vi "test_leadLag.vi"() -> ()   [LabVIEW 2019]
uses:
  <vilib>/Rock Robotics/WPI/ThirdParty/JAS_Junk/TrajLib/Util_GetTime.vi
  <vilib>/Rock Robotics/WPI/ThirdParty/JAS_Junk/TrajLib/Trajectory_Library.lvlib
panel:
  out "Waveform Chart":cluster{"Slide 2":dbl, "Output":dbl}(graph)
  in  "Lag Time Const (Sec)":dbl
  in  "Lead Time Const (Sec)":dbl
  in  "Enable":bool=TRUE
  out "Output":dbl(slide) scale=0.0..10.0
  in  "Input":dbl(slide) scale=0.0..10.0
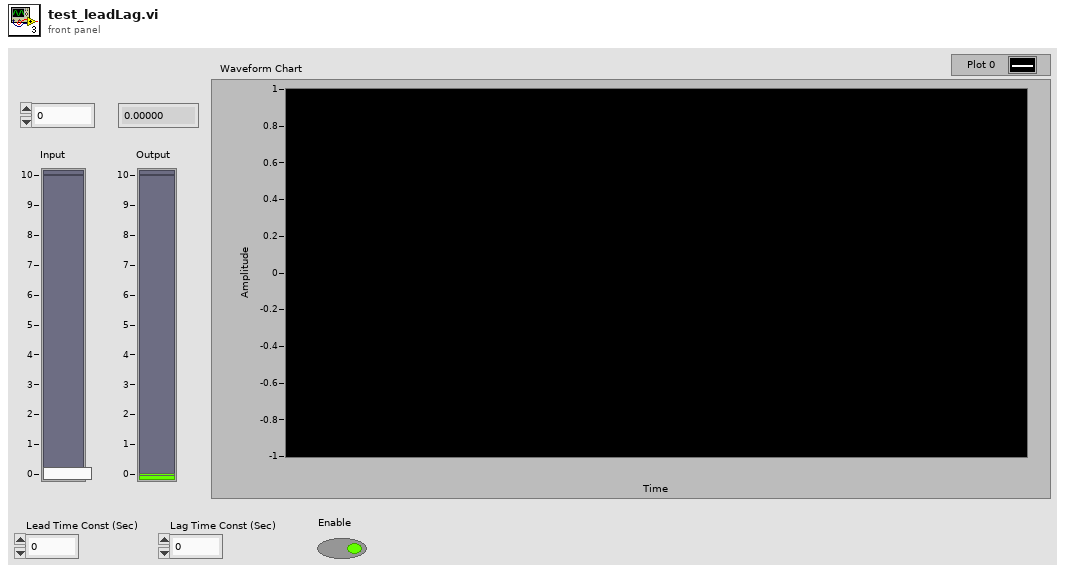
[diagram p1: front panel]
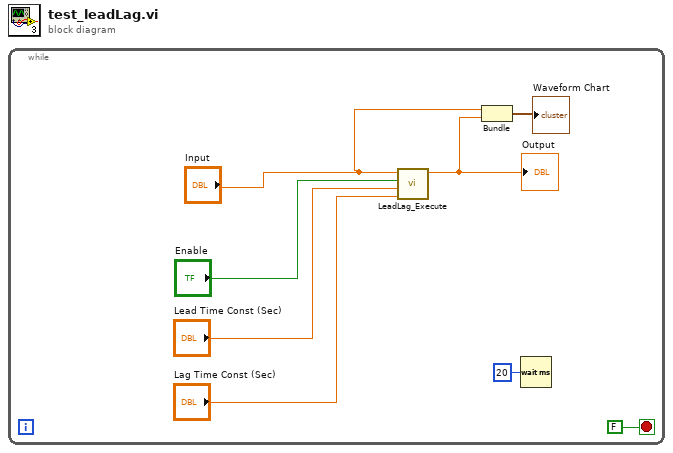
[diagram p0: block diagram]
diagram:
  n1 = while {
    stop <- FALSE stop-if-true
    n2 = call <vilib>:"LeadLag_Execute.vi"("Lag Time Const (Sec)"="Lag Time Const (Sec)", "Lead Time Const (Sec)"="Lead Time Const (Sec)", "Enable"="Enable", "Input"="Input") -> ("Output"=w1:dbl)  [unwired: 7 in]
    "Output" <- w1
    n3 = Bundle("Input"="Input", "Output"=w1) -> (→"Waveform Chart":cluster{"Input":dbl, "Output":dbl})  [unwired: 1 in]
    n4 = Wait (ms)(milliseconds to wait=u32 20) -> ()  [unwired: 1 out]
  }
